vi "TestResultGlo.vi"() -> ()   [LabVIEW 2020]
panel:
  in  "type":string
  in  "VC2_6":string
  in  "VC2_5":string
  in  "VC2_4":string
  in  "VC2_3":string
  in  "VC2_2":string
  in  "VC2_1":string
  in  "VC1_6":string
  in  "VC1_5":string
  in  "VC1_4":string
  in  "VC1_3":string
  in  "VC1_2":string
  in  "VC1_1":string
  in  "VC0_6":string
  in  "VC0_5":string
  in  "VC0_4":string
  in  "VC0_3":string
  in  "VC0_2":string
  in  "VC0_1":string
  in  "TC2_2":string
  in  "TC2_1":string
  in  "TC1_2":string
  in  "TC1_1":string
  in  "TC0_2":string
  in  "TC0_1":string
  in  "DcirP":string
  in  "DcirN":string
  in  "InsuN":string
  in  "InsuP":string
  in  "ACIR":string
  in  "OCV":string
  in  "ImageVers":string
  in  "tps_test":string
  in  "PASS":string
  in  "SoftVers":string
  in  "IniFileVers":string
  in  "date_start":string
  in  "SN":string
  in  "Operateur":string
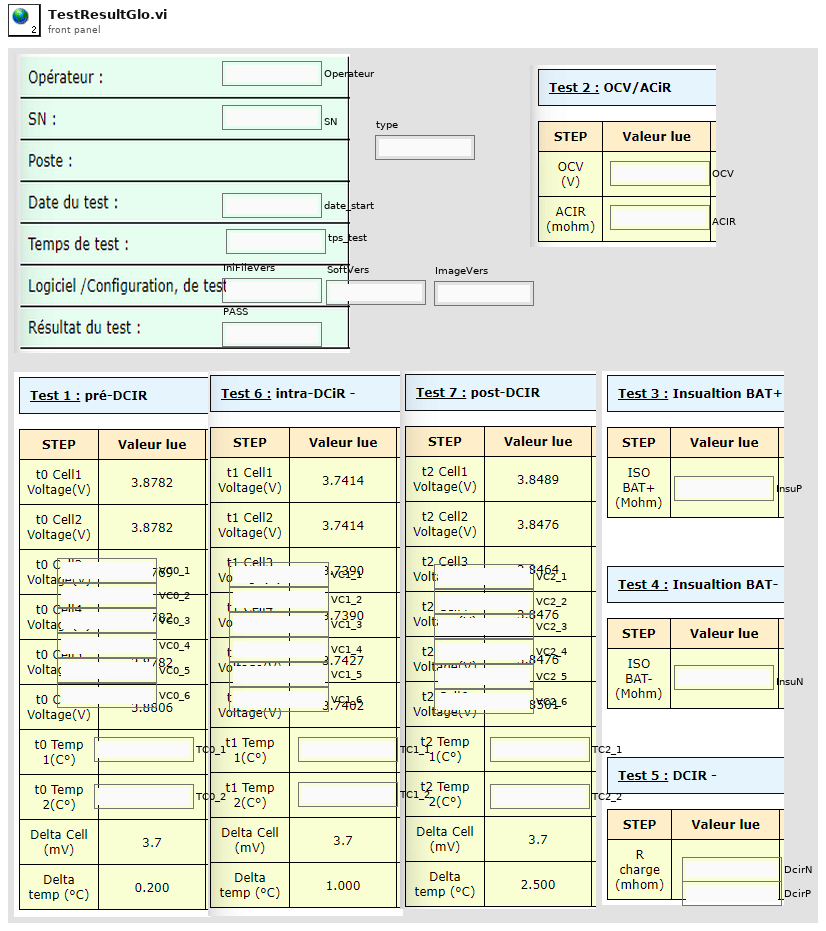
[diagram p1: front panel]
diagram:
